vi "Get Channel Settings.vi"(8 "error in":errorcluster, 11 "Node Ptr":T1 format="%.0x") -> (0 "error out":errorcluster, 2 "Channel Settings":T2, 3 "Node Ptr out":T1 format="%.0x")   [LabVIEW 2026]
uses:
  <vilib>/NI VeriStand/Custom Device API/Custom Device Item Ref.ctl
  Types/ChannelSettings.ctl
  NationalInstruments.VeriStand.SystemStorage
  <vilib>/NI VeriStand/Custom Device API/Custom Device API.lvlib
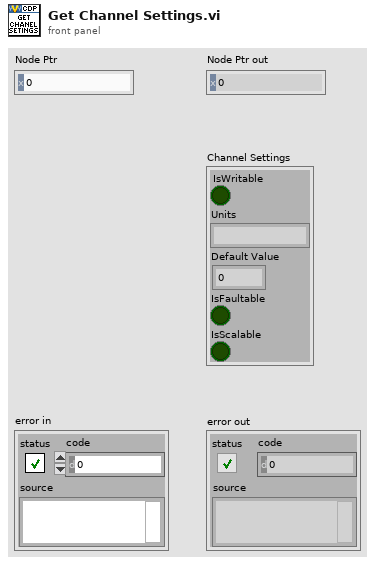
[diagram p1: front panel]
types:
  T1 = typedef "Custom Device API.lvlib/Custom Device Item Ref.ctl" = u64
  T2 = typedef "ChannelSettings.ctl" = cluster{"IsWritable":bool, "Units":string, "Default Value":dbl, "IsFaultable":bool, "IsScalable":bool}
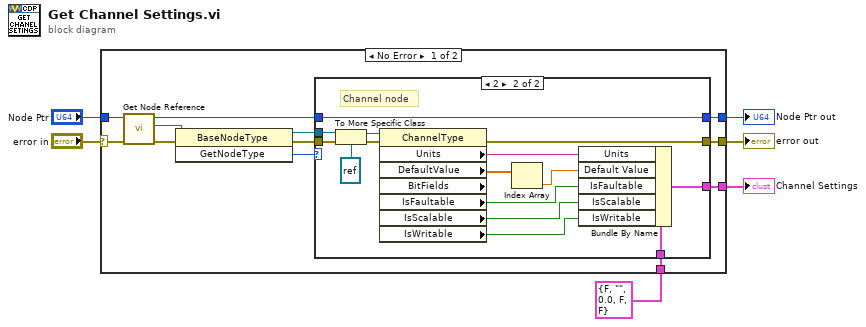
[diagram p0: block diagram]
diagram:
  n1 = case shown="No Error" "error in" {
    selector: "error in" -> [w18 w38]
    tunnel: "Node Ptr" -> [w17 w37]
    tunnel: [w11 w39] -> w5
    tunnel: T2 {"IsWritable"=FALSE, "Units"="", "Default Value"=0.0, "IsFaultable"=FALSE, "IsScalable"=FALSE} ("Channel Settings") -> [w10 w39]
    tunnel: [w9 w38] -> w2
    tunnel: [w7 w37] -> w1
    frame No Error {
      n2 = call "Get Node Reference.vi"("error in"=w18, "Node Ptr"=w17) -> ("error out"=w15:errorcluster, "BaseNodeType"=w16:refnum<k24>, "Node Ptr"=w8:T1)  [unwired: 6 in, 1 out]
      n3 = invoke class="BaseNodeType" method="GetNodeType"(reference=w16, error in=w15) -> (reference out=w12:refnum<k24>, error out=w13:errorcluster, "GetNodeType"=w14:i32)  [unwired: 1 in]
      n4 = case shown="2" w14 {
        tunnel: w13 -> [w20 w36]
        tunnel: w12 -> [_ w35]
        tunnel: [w21 w27] -> w11
        tunnel: w10 -> [w21 w24]
        tunnel: [w20 w23] -> w9
        tunnel: w8 -> [w19 w22]
        tunnel: [w19 w22] -> w7
        frame 0, Default {
        }
        frame 2 {
          # "Channel node"
          n5 = To More Specific Class(target class=refnum<k24> refnum ("reference"), reference=w35, error in=w36) -> (specific class reference=w33:refnum<k24>, error out=w32:errorcluster)
          n6 = property class="ChannelType" props=["Units", "DefaultValue", "BitFields", "IsFaultable", "IsScalable", "IsWritable"](reference=w33, error in=w32) -> (error out=w23:errorcluster, "Units"=w31:string, "DefaultValue"=w26:dbl[], "IsFaultable"=w30:bool, "IsScalable"=w29:bool, "IsWritable"=w28:bool)  [unwired: 2 out]
          n7 = Index Array(array=w26) -> (element=w25:dbl)  [unwired: 1 in]
          n8 = Bundle By Name(cluster=w24, "Units"=w31, "Default Value"=w25, "IsFaultable"=w30, "IsScalable"=w29, "IsWritable"=w28) -> (w27:T2)
        }
      }
    }
    frame Error {
    }
  }
  "Channel Settings" <- w5
  "error out" <- w2
  "Node Ptr out" <- w1
